vi "Status Monitor (SubVI).vi"(8 "error in":errorcluster, 11 "configuration file path":path) -> (0 "error out":errorcluster, 2 "New Status Message":bool, 3 "Module Carrier Status":T1)   [LabVIEW 2017, in "Status Monitor Library.lvlib"]
doc: "Use this template to build a producer/consumer design pattern. Use this template when you need to execute a process, such as data analysis, when a data source, such as a triggered acquisition, produces data at an uneven rate and you need to execute the process when the data becomes available."
uses:
  Status Monitor Library.lvlib
  Communications/Typedefs/DTACQ Module Carrier Status.ctl
  Communications/Typedefs/DTACQ Status--Enum.ctl
  Communications/Communications Library.lvlib
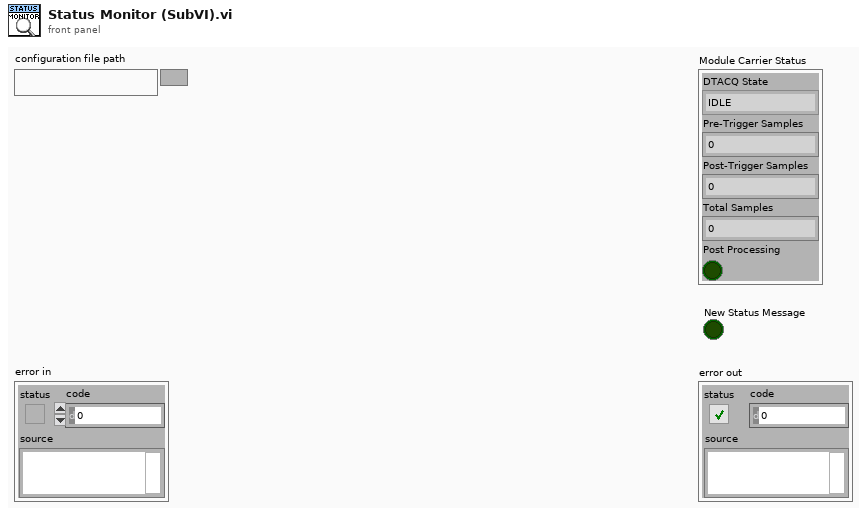
[diagram p1: front panel]
types:
  T1 = typedef "Communications Library.lvlib/DTACQ Module Carrier Status.ctl" = cluster{"DTACQ State":T2, "Pre-Trigger Samples":i32, "Post-Trigger Samples":i32, "Total Samples":i32, "Post Processing":bool}
  T2 = typedef "Communications Library.lvlib/DTACQ Status--Enum.ctl" = enum16{"IDLE", "ARM", "RUN_PRE-TRIGGER", "RUN_POST-TRIGGER", "POST_PROCESS", "CLEANUP"}
  T3 = typedef "Communications Library.lvlib/DTACQ Module Carrier Configuration--Cluster.ctl" = cluster{"Name":string, "IP":string, "Control Port":i32, "Timeout (ms)":i32, "Continuous Capture Port (Multiplexed)":i32, "Start HIL Shot Port":i32, "AWG Upload Port (Multiplexed)":i32, "Download Captured Data Port (Multiplexed)":i32, "Module Slots":i32, "Module Configurations":T4[]}
  T4 = typedef "Communications Library.lvlib/DTACQ Module Configuration--Cluster.ctl" = cluster{"Name":string, "Position":string, "Module Type":T5, "Control Port":i32, "Timeout (ms)":i32, "Channels":i32}
  T5 = typedef "Communications Library.lvlib/DTACQ Device Type--Enum.ctl" = enum16{"Carrier", "Analog In Module", "Analog Out Module", "Generic Module"}
  T6 = typedef "Communications Library.lvlib/DTACQ Connection Data--Cluster.ctl" = cluster{"Description":string, "Address":string, "Port":u16, "timeout (ms)":i32, "Termination Character":string, "TCP Connection Reference":refnum<k5>, "Open Connection":bool}
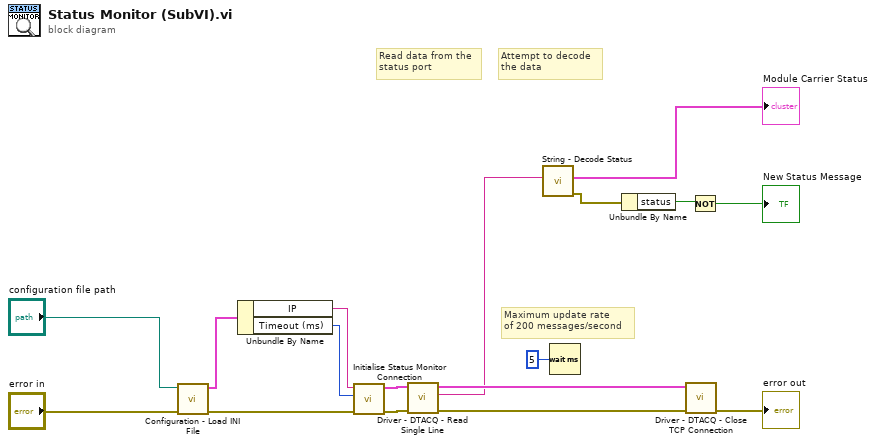
[diagram p0: block diagram]
diagram:
  # "Maximum update rate\nof 200 messages/second"
  # "Attempt to decode\nthe data"
  # "Read data from the\nstatus port"
  n1 = call "Configuration - Load INI File.vi"("error in"="error in", "configuration file path"="configuration file path") -> ("error out"=w10:errorcluster, "Carrier Configuration Out"=w12:T3)  [unwired: 8 in]
  n2 = Unbundle By Name(w12) -> ("IP"=w11:string, "Timeout (ms)"=w9:i32)
  n3 = call "Initialise Status Monitor Connection.vi"("error in"=w10, "timeout (ms)"=w9, "Address"=w11) -> ("error out"=w16:errorcluster, "Status Connection Out"=w17:T6)  [unwired: 7 in]
  n4 = call "Driver - DTACQ - Read Single Line.vi"("error in"=w16, "DTACQ Connection Data In"=w17) -> ("error out"=w15:errorcluster, "Read String"=w8:string, "DTACQ Connection Data Out"=w14:T6)  [unwired: 6 in, 1 out]
  n5 = call "String - Decode Status.vi"("Status Response String"=w8) -> ("error out"=w4:errorcluster, "Module Carrier Status"=→"Module Carrier Status":T1)  [unwired: 9 in]
  n6 = Wait (ms)(milliseconds to wait=u32 5) -> ()  [unwired: 1 out]
  n7 = Unbundle By Name(w4) -> ("status"=w3:bool)
  n8 = call "Driver - DTACQ - Close TCP Connection.vi"("error in"=w15, "DTACQ Connection Data In"=w14) -> ("error out"=→"error out":errorcluster)  [unwired: 8 in, 1 out]
  n9 = Not(x=w3) -> (.not. x?=→"New Status Message":bool)
